vi "controlGenerator.vi"(10 "ControlOutputPath":path, 11 "ComponentIDLFile":path) -> (0 "error out":errorcluster)   [LabVIEW 2016]
uses:
  IDLFile/IDLFile.lvclass
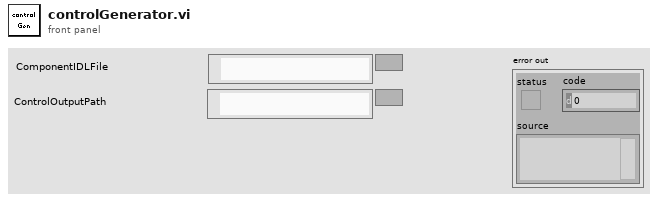
[diagram p1: front panel]
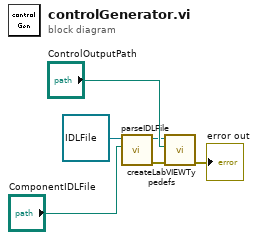
[diagram p0: block diagram]
diagram:
  n1 = call "parseIDLFile.vi"("idlFilepath"="ComponentIDLFile", "IDLFile in"=refnum<class "IDLFile.lvclass"> refnum ("IDLParser in")) -> ("error out"=w2:errorcluster, "IDLFile out"=w3:refnum<class "IDLFile.lvclass">)  [unwired: 8 in]
  n2 = call "createLabVIEWTypedefs.vi"("error in (no error)"=w2, "targetBasePath"="ControlOutputPath", "IDLFile in"=w3) -> ("error out"=→"error out":errorcluster)  [unwired: 7 in, 1 out]
